vi "VI_Tree.vi"   [LabVIEW 2017, in "GL860_Driver.lvlib"]
uses:
  GL860_Driver.lvlib
  GLdrv_Open_USB.vi
panel:
  # "Graphtec GL860\nLabVIEW Driver"
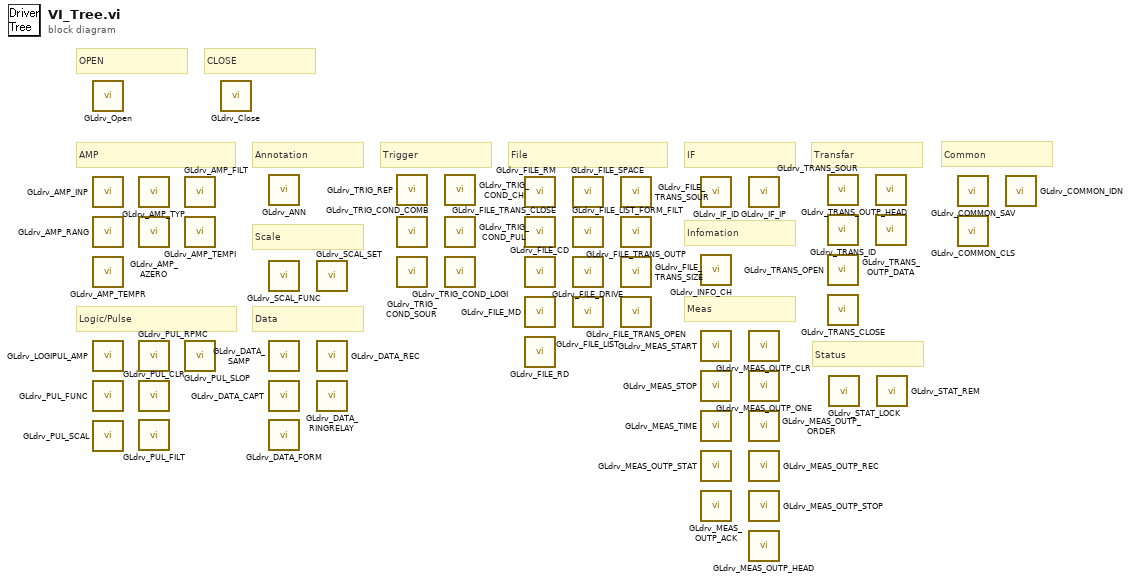
[diagram p0: block diagram]
diagram:
  # "Common"
  # "Status"
  # "Transfar"
  # "Meas"
  # "Infomation"
  # "IF"
  # "File"
  # "Trigger"
  # "Data"
  # "Scale"
  # "Annotation"
  # "CLOSE"
  # "OPEN"
  # "Logic/Pulse"
  # "AMP"
  n1 = call-poly "GLdrv_Open.vi"() -> ()  [unwired: 1 in, 15 out]
  n2 = call "GLdrv_AMP_INP.vi"() -> ()  [unwired: 5 in, 11 out]
  n3 = call "GLdrv_AMP_RANG.vi"() -> ()  [unwired: 5 in, 11 out]
  n4 = call "GLdrv_AMP_TEMPR.vi"() -> ()  [unwired: 13 in, 3 out]
  n5 = call "GLdrv_LOGIPUL_AMP.vi"() -> ()  [unwired: 5 in, 11 out]
  n6 = call "GLdrv_PUL_FUNC.vi"() -> ()  [unwired: 5 in, 11 out]
  n7 = call "GLdrv_PUL_SCAL.vi"() -> ()  [unwired: 8 in, 8 out]
  n8 = call "GLdrv_AMP_TYP.vi"() -> ()  [unwired: 3 in, 13 out]
  n9 = call "GLdrv_AMP_AZERO.vi"() -> ()  [unwired: 5 in, 11 out]
  n10 = call "GLdrv_PUL_RPMC.vi"() -> ()  [unwired: 5 in, 11 out]
  n11 = call "GLdrv_PUL_CLR.vi"() -> ()  [unwired: 3 in, 13 out]
  n12 = call "GLdrv_PUL_FILT.vi"() -> ()  [unwired: 13 in, 3 out]
  n13 = call "GLdrv_AMP_FILT.vi"() -> ()  [unwired: 5 in, 11 out]
  n14 = call "GLdrv_AMP_TEMPI.vi"() -> ()  [unwired: 13 in, 3 out]
  n15 = call "GLdrv_PUL_SLOP.vi"() -> ()  [unwired: 13 in, 3 out]
  n16 = call "GLdrv_Close.vi"() -> ()  [unwired: 2 in, 14 out]
  n17 = call "GLdrv_ANN.vi"() -> ()  [unwired: 13 in, 3 out]
  n18 = call "GLdrv_SCAL_FUNC.vi"() -> ()  [unwired: 5 in, 11 out]
  n19 = call "GLdrv_DATA_SAMP.vi"() -> ()  [unwired: 4 in, 12 out]
  n20 = call "GLdrv_DATA_CAPT.vi"() -> ()  [unwired: 5 in, 11 out]
  n21 = call "GLdrv_DATA_FORM.vi"() -> ()  [unwired: 4 in, 12 out]
  n22 = call "GLdrv_SCAL_SET.vi"() -> ()  [unwired: 5 in, 11 out]
  n23 = call "GLdrv_DATA_REC.vi"() -> ()  [unwired: 13 in, 3 out]
  n24 = call "GLdrv_DATA_RINGRELAY.vi"() -> ()  [unwired: 12 in, 4 out]
  n25 = call "GLdrv_TRIG_REP.vi"() -> ()  [unwired: 4 in, 12 out]
  n26 = call "GLdrv_TRIG_COND_COMB.vi"() -> ()  [unwired: 5 in, 11 out]
  n27 = call "GLdrv_TRIG_COND_SOUR.vi"() -> ()  [unwired: 7 in, 9 out]
  n28 = call "GLdrv_TRIG_COND_CH.vi"() -> ()  [unwired: 6 in, 10 out]
  n29 = call "GLdrv_TRIG_COND_PUL.vi"() -> ()  [unwired: 6 in, 10 out]
  n30 = call "GLdrv_TRIG_COND_LOGI.vi"() -> ()  [unwired: 6 in, 10 out]
  n31 = call "GLdrv_FILE_RM.vi"() -> ()  [unwired: 3 in, 13 out]
  n32 = call "GLdrv_FILE_TRANS_CLOSE.vi"() -> ()  [unwired: 2 in, 14 out]
  n33 = call "GLdrv_FILE_CD.vi"() -> ()  [unwired: 4 in, 12 out]
  n34 = call "GLdrv_FILE_MD.vi"() -> ()  [unwired: 3 in, 13 out]
  n35 = call "GLdrv_FILE_RD.vi"() -> ()  [unwired: 3 in, 13 out]
  n36 = call "GLdrv_FILE_SPACE.vi"() -> ()  [unwired: 2 in, 14 out]
  n37 = call "GLdrv_FILE_LIST_FORM_FILT.vi"() -> ()  [unwired: 5 in, 11 out]
  n38 = call "GLdrv_FILE_DRIVE.vi"() -> ()  [unwired: 2 in, 14 out]
  n39 = call "GLdrv_FILE_LIST.vi"() -> ()  [unwired: 2 in, 14 out]
  n40 = call "GLdrv_FILE_TRANS_SOUR.vi"() -> ()  [unwired: 4 in, 12 out]
  n41 = call "GLdrv_FILE_TRANS_OUTP.vi"() -> ()  [unwired: 5 in, 11 out]
  n42 = call "GLdrv_FILE_TRANS_SIZE.vi"() -> ()  [unwired: 2 in, 14 out]
  n43 = call "GLdrv_FILE_TRANS_OPEN.vi"() -> ()  [unwired: 2 in, 14 out]
  n44 = call "GLdrv_IF_ID.vi"() -> ()  [unwired: 4 in, 12 out]
  n45 = call "GLdrv_INFO_CH.vi"() -> ()  [unwired: 2 in, 14 out]
  n46 = call "GLdrv_MEAS_START.vi"() -> ()  [unwired: 2 in, 14 out]
  n47 = call "GLdrv_MEAS_STOP.vi"() -> ()  [unwired: 2 in, 14 out]
  n48 = call "GLdrv_MEAS_TIME.vi"() -> ()  [unwired: 2 in, 14 out]
  n49 = call "GLdrv_MEAS_OUTP_STAT.vi"() -> ()  [unwired: 11 in, 5 out]
  n50 = call "GLdrv_MEAS_OUTP_ACK.vi"() -> ()  [unwired: 13 in, 3 out]
  n51 = call "GLdrv_IF_IP.vi"() -> ()  [unwired: 4 in, 12 out]
  n52 = call "GLdrv_MEAS_OUTP_CLR.vi"() -> ()  [unwired: 2 in, 14 out]
  n53 = call "GLdrv_MEAS_OUTP_ONE.vi"() -> ()  [unwired: 2 in, 14 out]
  n54 = call "GLdrv_MEAS_OUTP_ORDER.vi"() -> ()  [unwired: 13 in, 3 out]
  n55 = call "GLdrv_MEAS_OUTP_REC.vi"() -> ()  [unwired: 2 in, 14 out]
  n56 = call "GLdrv_MEAS_OUTP_STOP.vi"() -> ()  [unwired: 2 in, 14 out]
  n57 = call "GLdrv_MEAS_OUTP_HEAD.vi"() -> ()  [unwired: 2 in, 14 out]
  n58 = call "GLdrv_TRANS_SOUR.vi"() -> ()  [unwired: 5 in, 11 out]
  n59 = call "GLdrv_TRANS_ID.vi"() -> ()  [unwired: 13 in, 3 out]
  n60 = call "GLdrv_TRANS_OPEN.vi"() -> ()  [unwired: 2 in, 14 out]
  n61 = call "GLdrv_TRANS_CLOSE.vi"() -> ()  [unwired: 2 in, 14 out]
  n62 = call "GLdrv_STAT_LOCK.vi"() -> ()  [unwired: 4 in, 12 out]
  n63 = call "GLdrv_TRANS_OUTP_HEAD.vi"() -> ()  [unwired: 2 in, 14 out]
  n64 = call "GLdrv_TRANS_OUTP_DATA.vi"() -> ()  [unwired: 5 in, 11 out]
  n65 = call "GLdrv_STAT_REM.vi"() -> ()  [unwired: 3 in, 13 out]
  n66 = call "GLdrv_COMMON_SAV.vi"() -> ()  [unwired: 14 in, 2 out]
  n67 = call "GLdrv_COMMON_CLS.vi"() -> ()  [unwired: 14 in, 2 out]
  n68 = call "GLdrv_COMMON_IDN.vi"() -> ()  [unwired: 13 in, 3 out]
